vi "Review Result.vi"(0 "SA Path in":refnum<class "SA Abstract Path.lvclass">, 11 "error in (no error)":errorcluster) -> (4 "SA Path out":refnum<class "SA Abstract Path.lvclass">, 6 "Response":string, 15 "error out":errorcluster)   [LabVIEW 2023, in "RFFixtureCharact.Public.lvlib" / "SA Abstract Path.lvclass"]
uses:
  SA Abstract Path.lvclass
  <vilib>/Utility/error.llb/Trim Whitespace One-Sided.vi
  Scalar Path/Scalar Path.lvclass
  Common/RFCalAndFixtureCharact.Common.lvlib
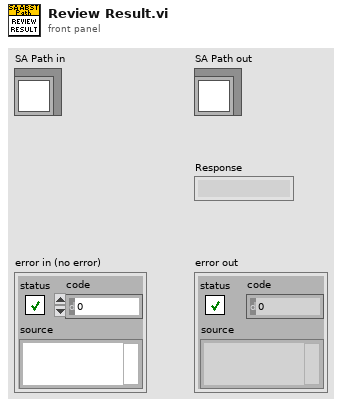
[diagram p1: front panel]
types:
  T1 = typedef "RFFixtureCharact.Public.lvlib/Scalar Path.lvclass/Scalar Charact Result.ctl" = cluster{"Port Power":dbl, "Reference Level":dbl, "Frequency":dbl, "Path Gain":dbl, "Out Of Limit":bool}
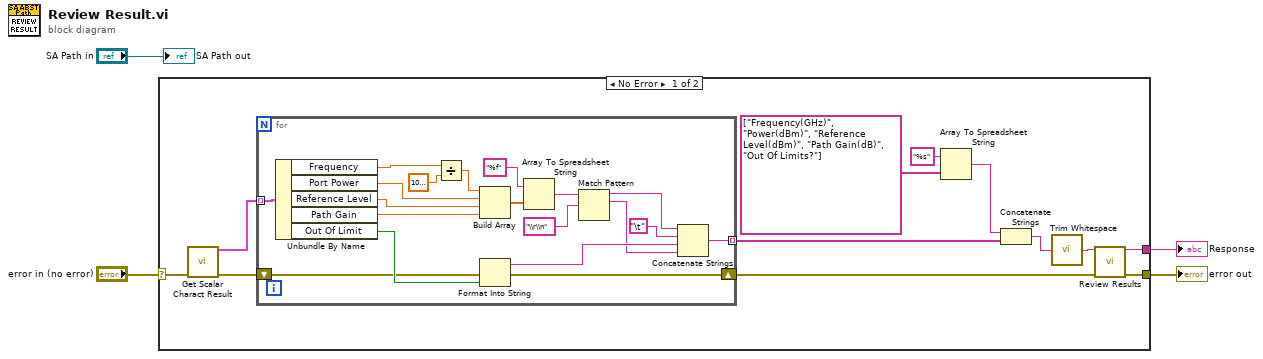
[diagram p0: block diagram]
diagram:
  n1 = case shown="No Error" "error in (no error)" {
    selector: "error in (no error)" -> [w12 w36]
    tunnel: [w13 w36] -> w1
    tunnel: [w14 _] -> w2
    frame No Error {
      n2 = call "Get Scalar Charact Result.vi"("error in (no error)"=w12) -> ("Charact result"=w16:T1[], "error out"=w11:errorcluster)  [unwired: 13 in]
      n3 = for {
        tunnel: w16 -> [w35] mode=indexing
        tunnel: [w29] -> w15 mode=indexing
        shift-right: [w24] -> w10
        shift-left: w11 -> [w25]
        n4 = Unbundle By Name(w35) -> ("Frequency"=w17:dbl, "Port Power"=w34:dbl, "Reference Level"=w18:dbl, "Path Gain"=w19:dbl, "Out Of Limit"=w31:bool)
        n5 = Divide(x=w17, y=1000000000.0) -> (x/y=w20:dbl)
        n6 = Build Array(w20, w34, w18, w19) -> (w33:dbl[])
        n7 = Format Into String(error in=w25, w31) -> (resulting string=w30:string, error out=w24:errorcluster)  [unwired: 2 in]
        n8 = Array To Spreadsheet String(array=w33, 3:"%f" ("format string")) -> (spreadsheet string=w27:string)  [unwired: 1 in]
        n9 = Match Pattern(string=w27, regular expression="\\r\\n") -> (before substring=w26:string, match substring=w22:string)  [unwired: 1 in, 2 out]
        n10 = Concatenate Strings(w26, "\t", w30, w22) -> (w29:string)
      }
      n11 = Array To Spreadsheet String(array=string[] ["Frequency(GHz)", "Power(dBm)", "Reference Level(dBm)", "Path Gain(dB)", "Out Of Limits?"], 3:"%s" ("format string")) -> (spreadsheet string=w5:string)  [unwired: 1 in]
      n12 = Concatenate Strings(w5, w15) -> (w9:string)
      n13 = call <vilib>:"Trim Whitespace.vi"("string"=w9) -> ("trimmed string"=w8:string)  [unwired: 1 in]
      n14 = call "Review Results.vi"("Cal Results"=w8, "error in (no error)"=w10) -> ("Response"=w14:string, "error out"=w13:errorcluster)  [unwired: 12 in]
    }
    frame Error {
    }
  }
  "error out" <- w1
  "Response" <- w2
  "SA Path out" <- "SA Path in"
